vi "Call Easing Function Dynamically.vi"(8 "error in":errorcluster, 11 "Display State In":T1={"Numeric"=0.0, "Array of Button References"=[], "Space Between Menu Buttons"=0, "Number of Menu Buttons"=0, "Array of Button Names"=[], "Most Recent Vertical Position"=0, "This VI"=refnum, "Current Action"=enum."Not Moving", "Most Recent Distance Traveled"=0, "Method"=enum."Move Up", "Data In"=0} caption="State") -> (0 "error out":errorcluster, 3 "Display State Out":T1={"Numeric"=0.0, "Array of Button References"=[], "Space Between Menu Buttons"=0, "Number of Menu Buttons"=0, "Array of Button Names"=[], "Most Recent Vertical Position"=0, "This VI"=refnum, "Current Action"=enum."Not Moving", "Most Recent Distance Traveled"=0, "Method"=enum."Move Up", "Data In"=0} caption="State")   [LabVIEW 2011, in "Sliding Menu Library.lvlib" / "Sliding Menu XControl.xctl"]
uses:
  Sliding Menu XControl.xctl
  Sliding Menu State.ctl
  Menu Button Library/Menu Button xControl/Menu Button xControl.xctl
  Sliding Menu SubVIs/Sliding Menu Type Definitions/Current User Action.ctl
  Sliding Menu Methods.ctl
  Sliding Menu Data.ctl
  Sliding Menu Library.lvlib
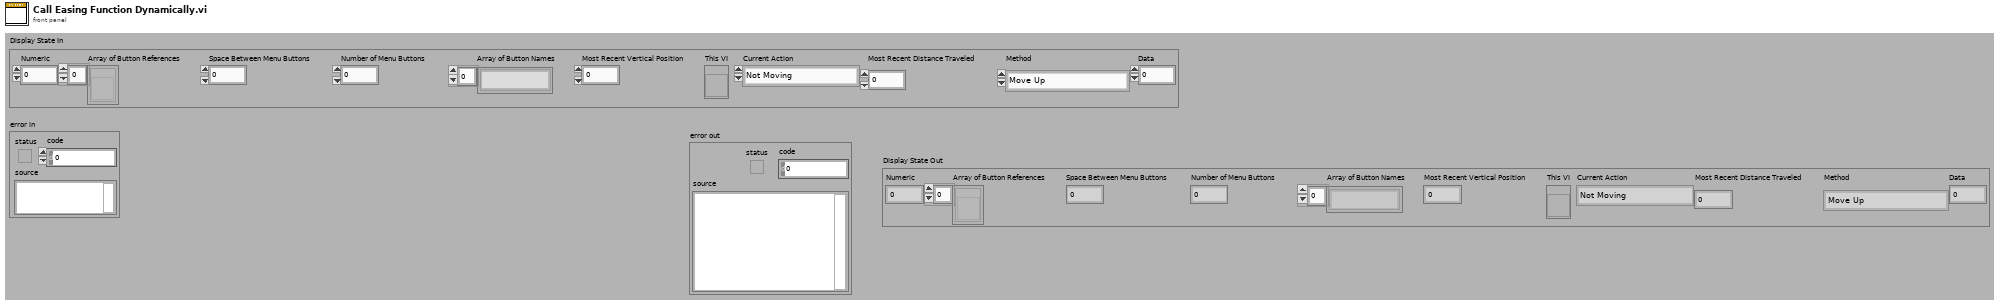
[diagram p1: front panel]
types:
  T1 = typedef "Sliding Menu Library.lvlib/Sliding Menu XControl.xctl/Sliding Menu State.ctl" = cluster{"Numeric":dbl, "Array of Button References":refnum<vi>[], "Space Between Menu Buttons":i32, "Number of Menu Buttons":i32, "Array of Button Names":string[], "Most Recent Vertical Position":i32, "This VI":refnum<vi>, "Current Action":T2, "Most Recent Distance Traveled":i32, "Method":T3, "Data In":T4}
  T2 = typedef "Sliding Menu Library.lvlib/Current User Action.ctl" = enum16{"Not Moving", "Mouse Down", "Mouse Up No Dragging", "Bounce Up Needed", "Bounce Down Needed", "Dragging", "Easing"}
  T3 = typedef "Sliding Menu Methods.ctl" = enum16{"Resize", "Move Up", "Move Down", "Move to 0"}
  T4 = typedef "Sliding Menu Library.lvlib/Sliding Menu XControl.xctl/Sliding Menu Data.ctl" = i32
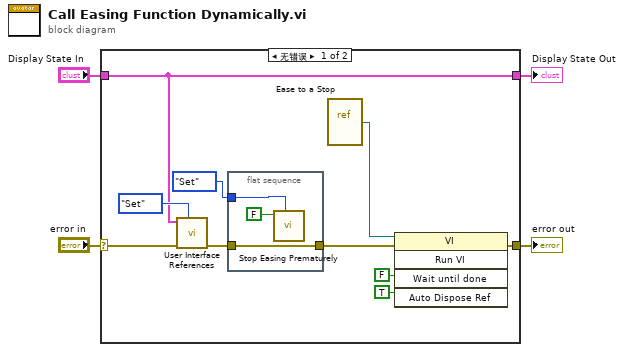
[diagram p0: block diagram]
diagram:
  n1 = case shown="无错误" "error in" {
    selector: "error in" -> [w11 w18]
    tunnel: [w9 w18] -> w1
    tunnel: "Display State In" -> [w10 w19]
    tunnel: [w10 w19] -> w2
    frame No Error {
      n2 = call "User Interface References.vi"("Set or Get Value"=enum16{"Set", "Get"}."Set", "error in"=w11, "Display State In"=w10) -> ("error out"=w12:errorcluster)  [unwired: 7 in, 1 out]
      n3 = flat-sequence {
        tunnel: enum16{"Set", "Get"}."Set" ("Set or Get Value") -> [w16]
        tunnel: w12 -> [w15]
        tunnel: [w15] -> w5
        frame #0 {
          n4 = call "Stop Easing Prematurely.vi"("Set or Get Value"=w16, "Stop?"=FALSE) -> ()  [unwired: 9 in, 1 out]
        }
      }
      n5 = vi-ref "Ease to a Stop.vi"() -> (w6:refnum<vi>)
      n6 = invoke class="VI" method="Run VI"(reference=w6, error in=w5, "Wait until done"=FALSE ("Wait Until Done"), "Auto Dispose Ref"=TRUE ("Auto Dispose Reference")) -> (error out=w9:errorcluster)  [unwired: 1 in, 4 out]
    }
    frame Error {
    }
  }
  "error out" <- w1
  "Display State Out" <- w2
